vi "writeToXML.vi"(8 "error in (no error)":errorcluster, 10 "ClassLabel":string, 11 "Rotator in":refnum<class "Rotator.lvclass">) -> (0 "error out":errorcluster, 2 "XML out":string, 3 "Rotator out":refnum<class "Rotator.lvclass">)   [LabVIEW 2014, in "TCSDataDefinitions.lvlib" / "TCSCommand.lvlib" / "TargetConfiguration.lvlib" / "Rotator.lvclass"]
uses:
  Rotator.lvclass
  <userlib>/Common/UnitsAndXML/FlattenItemWithUnitToXML/FlattenPlaneAngleToXML/PlaneAngleUnit.ctl
  Rotator.lvclass/Rotator.ctl
  <userlib>/Common/UnitsAndXML/UnitsAndXML.lvlib
  <userlib>/Common/XML/XMLGenerator/XMLGenerator.lvclass
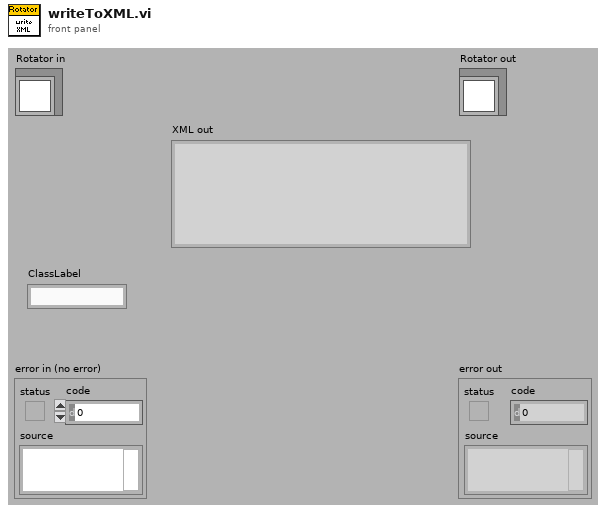
[diagram p1: front panel]
types:
  T1 = typedef "UnitsAndXML.lvlib/PlaneAngleUnit.ctl" = enum16{"rad", "deg", "'", "\""}
  T2 = typedef "TCSDataDefinitions.lvlib/TCSCommand.lvlib/RotatorFrameValues.ctl" = enum16{"Target", "Fixed"}
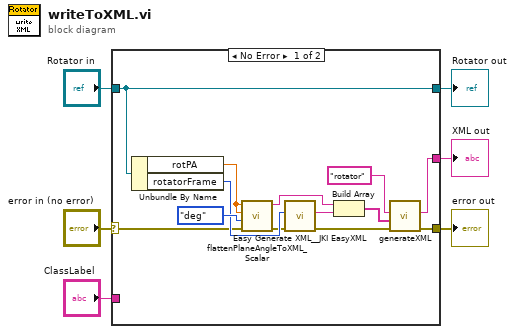
[diagram p0: block diagram]
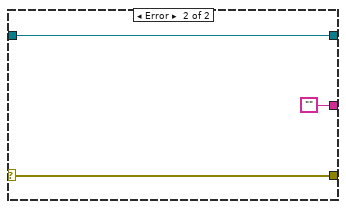
[diagram p2: hidden frame]
diagram:
  n1 = case shown="No Error" "error in (no error)" {
    selector: "error in (no error)" -> [w14 w22]
    tunnel: [w7 w22] -> w5
    tunnel: [w19 w21] -> w3
    tunnel: "Rotator in" -> [w19 w21]
    tunnel: [w8 ""] -> w2
    tunnel: "ClassLabel" -> [_ _]
    frame No Error {
      n2 = Unbundle By Name(w19) -> ("rotPA"=w18:dbl[unit], "rotatorFrame"=w16:T2)
      n3 = call <userlib>:"flattenPlaneAngleToXML_Scalar.vi"("error in (no error)"=w14, "planeAngleUnitInXML"=PlaneAngleUnit."deg", "planeAngleAgain"=w18, "planeAngle"=w18) -> ("error out"=w15:errorcluster, "xmlString"=w11:string)  [unwired: 6 in]
      n4 = call <vilib>:"Easy Generate XML__JKI EasyXML.vi"("error in (no error)"=w15, "LabVIEW Data"=w16) -> ("error out"=w13:errorcluster, "XML String"=w12:string)  [unwired: 8 in]
      n5 = Build Array(w11, w12) -> (w10:string[])
      n6 = call <userlib>:"generateXML.vi"("error in"=w13, "childrenXML"=w10, "elementName"="rotator" ("Class Label")) -> ("error out"=w7:errorcluster, "XML out"=w8:string)  [unwired: 6 in, 1 out]
    }
    frame Error {
    }
  }
  "error out" <- w5
  "Rotator out" <- w3
  "XML out" <- w2
